vi "DSF.Shared.Configuration.JSON.Read File.vi"(8 "error in (no error)":errorcluster, 10 "path":path, 11 "JSON Configuration in":refnum<class "DSF.Shared.Configuration.JSON.lvclass">) -> (0 "error out":errorcluster, 1 "json string":string, 3 "JSON Configuration out":refnum<class "DSF.Shared.Configuration.JSON.lvclass">)   [LabVIEW 2017, in "DSF.Shared.lvlib" / "DSF.Shared.Configuration.JSON.lvclass"]
uses:
  DSF.Shared.Configuration.JSON.lvclass
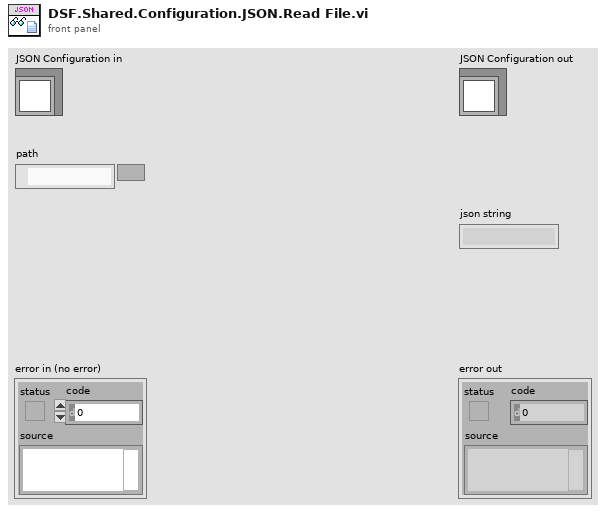
[diagram p1: front panel]
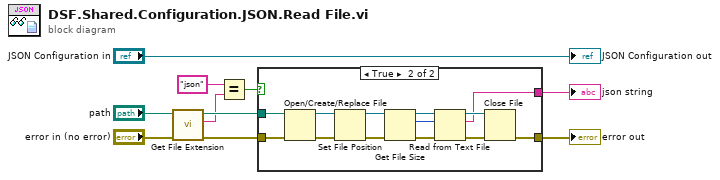
[diagram p0: block diagram]
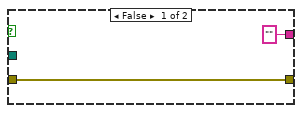
[diagram p2: hidden frame]
diagram:
  n1 = call <vilib>:"Get File Extension.vi"("error in (no error)"="error in (no error)", "file"="path") -> ("error out"=w5:errorcluster, "lowercase file extension"=w3:string, "dup file"=w4:path)  [unwired: 5 in, 2 out]
  n2 = Equal?(x="json", y=w3) -> (x = y?=w1:bool)
  n3 = case shown="True" w1 {
    tunnel: ["" w16] -> w9
    tunnel: [w12 w15] -> w8
    tunnel: w5 -> [w12 w14]
    tunnel: w4 -> [_ w13]
    frame False {
    }
    frame True {
      n4 = Open/Create/Replace File(file path (use dialog)=w13, error in=w14) -> (refnum out=w25:refnum<file>, error out=w24:errorcluster)  [unwired: 4 in, 1 out]
      n5 = Set File Position(refnum=w25, error in=w24) -> (refnum out=w23:refnum<file>, error out=w22:errorcluster)  [unwired: 2 in]
      n6 = Get File Size(file=w23, error in=w22) -> (refnum out=w21:refnum<file>, size (in bytes)=w20:i64, 0:w19:errorcluster)
      n7 = Read from Text File(file (use dialog)=w21, count=w20, error in=w19) -> (refnum out=w18:refnum<file>, text=w16:string, error out=w17:errorcluster)  [unwired: 1 in, 1 out]
      n8 = Close File(refnum=w18, error in=w17) -> (error out=w15:errorcluster)  [unwired: 1 out]
    }
  }
  "error out" <- w8
  "json string" <- w9
  "JSON Configuration out" <- "JSON Configuration in"
